vi "invert_and_blank.vi"(9 "zeroOutput":bool, 10 "invert":bool, 11 "input":i16) -> (3 "output":i16)   [LabVIEW 2016]
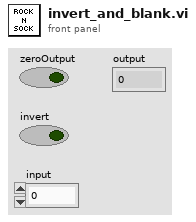
[diagram p1: front panel]
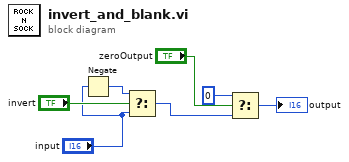
[diagram p0: block diagram]
diagram:
  n1 = Negate(x="input") -> (-x=w5:i16)
  n2 = Select(t=w5, s="invert", f="input") -> (s? t:f=w6:i16)
  n3 = Select(t=i16 0, s="zeroOutput", f=w6) -> (s? t:f=→"output":i16)
